vi "PTSequencer.obj params 2 byte array.vi"(2 "method parameters":T2(array[cluster])) -> (16 "byteArray out":T1)   [LabVIEW 2014, in "PTSequencer.lvlib"]
uses:
  PTSequencer.lvlib
  CS_Core/CSSystem/CoreDefs/CoreDefs.rawDataType.ctl
  CS_Core/CSSystem/CoreLib/CoreLib.string 2 byte array.vi
  CS_Core/CSSystem/CoreLib/CoreLib.int 2 byte array.vi
  CS_Core/CSSystem/CoreLib/CoreLib.int array 2 byte array.vi
  CS_Core/CSSystem/CoreLib/CoreLib.short 2 byte array.vi
  CS_Core/CSSystem/CoreLib/CoreLib.short array 2 byte array.vi
  CS_Core/CSSystem/CoreLib/CoreLib.double 2 byte array.vi
  CS_Core/CSSystem/CoreLib/CoreLib.float 2 byte array.vi
  CS_Core/CSSystem/CoreLib/CoreLib.double array 2 byte array.vi
  CS_Core/CSSystem/CoreLib/CoreLib.float array 2 byte array.vi
  CS_Core/CSSystem/CoreLib/CoreLib.lvlib
  _common/PTUtils/PTUtils.lvlib
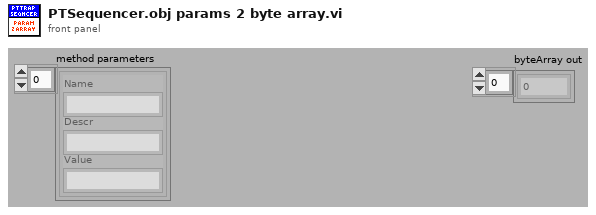
[diagram p1: front panel]
types:
  T1 = typedef "CoreDefs.rawDataType.ctl" = i8[]
  T2 = cluster{"Name":string, "Descr":string, "Value":string}[]
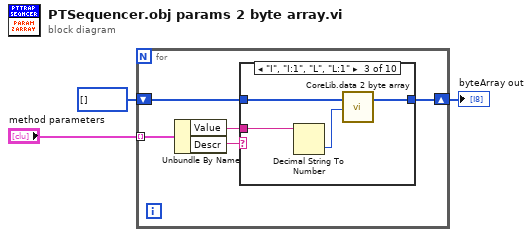
[diagram p0: block diagram]
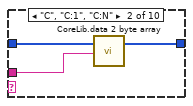
[diagram p3: hidden frame]
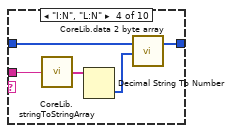
[diagram p4: hidden frame]
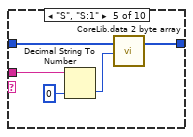
[diagram p5: hidden frame]
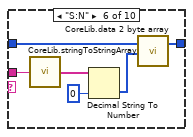
[diagram p6: hidden frame]
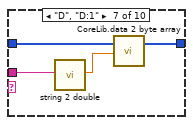
[diagram p7: hidden frame]
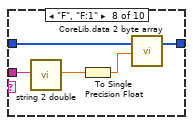
[diagram p8: hidden frame]
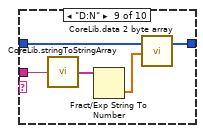
[diagram p9: hidden frame]
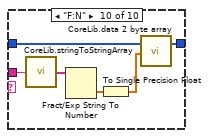
[diagram p10: hidden frame]
diagram:
  n1 = for {
    tunnel: "method parameters" -> [w8] mode=indexing
    shift-right: [w5] -> w1
    shift-left: T1 [] ("byteArray out") -> [w4]
    n2 = Unbundle By Name(w8) -> ("Value"=w6:string, "Descr"=w7:string)
    n3 = case shown="\"I\", \"I:1\", \"L\", \"L:1\"" w7 {
      tunnel: w6 -> [_ w12 w15 w20 w23 w28 w36 w41 w46 w52]
      tunnel: [w9 w11 w13 w17 w24 w30 w33 w39 w42 w49] -> w5
      tunnel: w4 -> [w9 w10 w16 w18 w25 w31 w34 w40 w44 w50]
      frame Default {
      }
      frame "C", "C:1", "C:N" {
        n4 = call-poly "CoreLib.data 2 byte array.vi"("byteArray"=w10, "string"=w12) -> ("byteArray out"=w11:T1)  [unwired: 17 in]
      }
      frame "I", "I:1", "L", "L:1" {
        n5 = Decimal String To Number(string=w15) -> (number=w14:i32)  [unwired: 2 in, 1 out]
        n6 = call-poly "CoreLib.data 2 byte array.vi"("byteArray"=w16, "i32"=w14) -> ("byteArray out"=w13:T1)  [unwired: 17 in]
      }
      frame "I:N", "L:N" {
        n7 = call "CoreLib.stringToStringArray.vi"("String"=w20) -> ("Array"=w19:string[])
        n8 = Decimal String To Number(string=w19) -> (number=w21:i32[])  [unwired: 2 in, 1 out]
        n9 = call-poly "CoreLib.data 2 byte array.vi"("byteArray"=w18, "[i32]"=w21) -> ("byteArray out"=w17:T1)  [unwired: 17 in]
      }
      frame "S", "S:1" {
        n10 = Decimal String To Number(string=w23, default (0L)=i16 0 ("default (0 I32)")) -> (number=w26:i16)  [unwired: 1 in, 1 out]
        n11 = call-poly "CoreLib.data 2 byte array.vi"("byteArray"=w25, "i16"=w26) -> ("byteArray out"=w24:T1)  [unwired: 17 in]
      }
      frame "S:N" {
        n12 = call "CoreLib.stringToStringArray.vi"("String"=w28) -> ("Array"=w27:string[])
        n13 = Decimal String To Number(string=w27, default (0L)=i16 0 ("default (0 I32)")) -> (number=w32:i16[])  [unwired: 1 in, 1 out]
        n14 = call-poly "CoreLib.data 2 byte array.vi"("byteArray"=w31, "[i16]"=w32) -> ("byteArray out"=w30:T1)  [unwired: 17 in]
      }
      frame "D", "D:1" {
        n15 = call "string 2 double.vi"("string"=w36) -> ("number"=w35:dbl)  [unwired: 15 in, 3 out]
        n16 = call-poly "CoreLib.data 2 byte array.vi"("byteArray"=w34, "f64"=w35) -> ("byteArray out"=w33:T1)  [unwired: 17 in]
      }
      frame "F", "F:1" {
        n17 = call "string 2 double.vi"("string"=w41) -> ("number"=w38:dbl)  [unwired: 15 in, 3 out]
        n18 = To Single Precision Float(number=w38) -> (single precision float=w37:sgl)
        n19 = call-poly "CoreLib.data 2 byte array.vi"("byteArray"=w40, "f32"=w37) -> ("byteArray out"=w39:T1)  [unwired: 17 in]
      }
      frame "D:N" {
        n20 = call "CoreLib.stringToStringArray.vi"("String"=w46) -> ("Array"=w45:string[])
        n21 = Fract/Exp String To Number(string=w45) -> (number=w43:dbl[])  [unwired: 3 in, 1 out]
        n22 = call-poly "CoreLib.data 2 byte array.vi"("byteArray"=w44, "[d64]"=w43) -> ("byteArray out"=w42:T1)  [unwired: 17 in]
      }
      frame "F:N" {
        n23 = call "CoreLib.stringToStringArray.vi"("String"=w52) -> ("Array"=w51:string[])
        n24 = Fract/Exp String To Number(string=w51) -> (number=w48:dbl[])  [unwired: 3 in, 1 out]
        n25 = To Single Precision Float(number=w48) -> (single precision float=w47:sgl[])
        n26 = call-poly "CoreLib.data 2 byte array.vi"("byteArray"=w50, "[f32]"=w47) -> ("byteArray out"=w49:T1)  [unwired: 17 in]
      }
    }
  }
  "byteArray out" <- w1
